vi "Prepare SQL Command.vi"   [LabVIEW 2023, in "SQLite DB Operator.lvclass"]
uses:
  SQLite DB Operator.lvclass
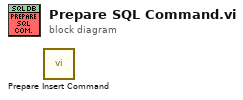
[diagram p0: block diagram]
diagram:
  n1 = call "Prepare Insert Command.vi"() -> ()  [unwired: 10 in, 2 out]
